vi "fr_ctrl.vi"(5 "amount":dbl, 7 "target":dbl, 10 "enable":i32, 11 "reset":i32) -> (4 "target / fr_actual":dbl, 6 "fr_actual":dbl)   [LabVIEW 2015]
uses:
  BERTTA.dll
panel:
  out "params3":i32
  out "params2":i32
  out "params1":i32
  out "params0":i32
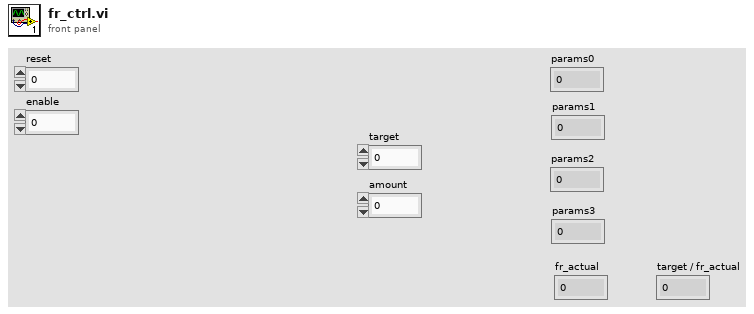
[diagram p1: front panel]
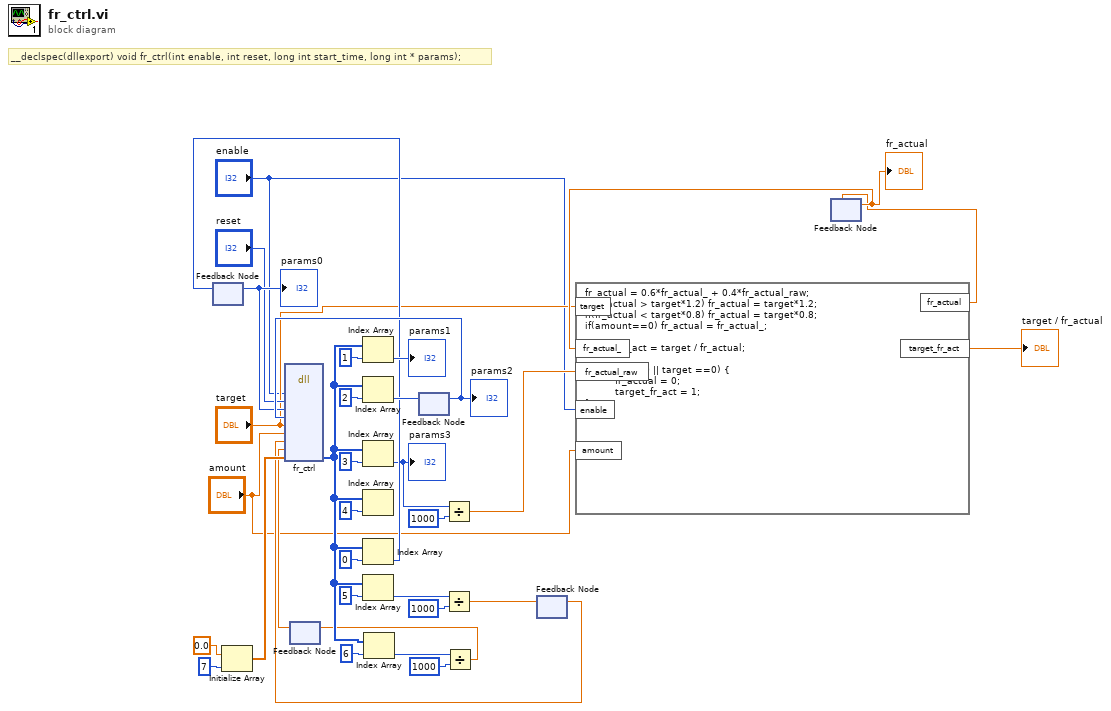
[diagram p0: block diagram]
diagram:
  # "__declspec(dllexport) void fr_ctrl(int enable, int reset, long int start_time, long int * params);"
  n1 = feedback #1() -> (w24:i32)  [unwired: 1 in]
  "params0" <- w24
  n2 = Initialize Array(0.0 ("element"), 7 ("dimension size")) -> (w32:dbl[])
  n3 = feedback #2() -> (w8:dbl)  [unwired: 1 in]
  n4 = feedback #3() -> (w26:i32)  [unwired: 1 in]
  "params2" <- w26
  n5 = feedback #4() -> (w14:dbl)  [unwired: 1 in]
  n6 = dll-call lib="C:/Users/shresplab/OneDrive - Kemira Oyj/Documents/Visual Studio 2017/Projects/Bertta/BERTTA/x64/Debug/BERTTA.dll" fn="fr_ctrl"("enable"="enable", "reset"="reset", "last_time"=w24, "elapsed_last"=w26, "target"="target", "amount"="amount", "amount_last"=w14, "fr_actual_last"=w8, "params"=w32) -> ("params"=w10:i32[])  [unwired: 12 in, 2 out]
  n7 = Index Array(array=w10, index=1) -> (element=→"params1":i32)
  n8 = Index Array(array=w10, index=2) -> (element=w27:i32)
  n9 = Index Array(array=w10, index=3) -> (element=w21:i32)
  "params3" <- w21
  n10 = Index Array(array=w10, index=4) -> ()  [unwired: 1 out]
  n11 = Index Array(array=w10, index=0) -> (element=w25:i32)
  n12 = feedback-in #1(w25) -> ()
  n13 = Index Array(array=w10, index=5) -> (element=w17:i32)
  n14 = Index Array(array=w10, index=6) -> (element=w12:i32)
  n15 = feedback-in #3(w27) -> ()
  n16 = Divide(x=w21, y=1000) -> (x/y=w7:dbl)
  n17 = Divide(x=w17, y=1000) -> (x/y=w15:dbl)
  n18 = Divide(x=w12, y=1000) -> (x/y=w9:dbl)
  n19 = feedback-in #2(w9) -> ()
  n20 = feedback-in #4(w15) -> ()
  n21 = feedback #5() -> (w6:dbl)  [unwired: 1 in]
  "fr_actual" <- w6
  n22 = formula code="fr_actual = 0.6*fr_actual_ + 0.4*fr_actual_raw;\nif(fr_actual > target*1.2) fr_actual = target*1.2;\nif(fr_actual < target*0.8) fr_actual = target*0.8;\nif(amount==0) fr_actual = fr_actual_;\n\ntarget_fr_act = target / fr_actual;\n\nif(enable==0 || target ==0) {\n          fr_actual = 0;\n          target_fr_act = 1;\n}"("fr_actual_raw"=w7, "fr_actual_"=w6, "target"="target", "enable"="enable", "amount"="amount") -> ("fr_actual"=w3:dbl, "target_fr_act"=→"target / fr_actual":dbl)
  n23 = feedback-in #5(w3) -> ()
